vi "SolveFastPath.vi"(8 "error in (no error)":errorcluster, 11 "RouteTree in":refnum<class "RouteTree.lvclass">) -> (0 "error out":errorcluster, 2 "greedy Path":T1[](array[typedef]), 3 "RouteTree out":refnum<class "RouteTree.lvclass">)   [LabVIEW 2010, in "RouteTree.lvclass"]
uses:
  RouteTree.lvclass
  Waypoint/point.ctl
  Waypoint/Waypoint.lvclass
  Tree/Tree.lvclass
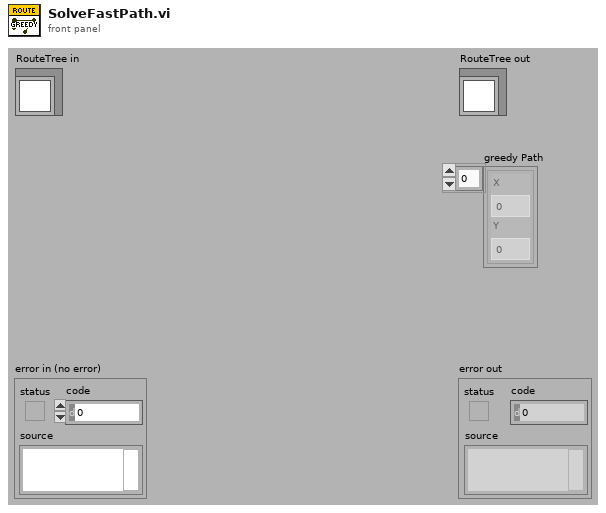
[diagram p1: front panel]
types:
  T1 = typedef "Waypoint.lvclass/point.ctl" = cluster{"X":dbl, "Y":dbl}
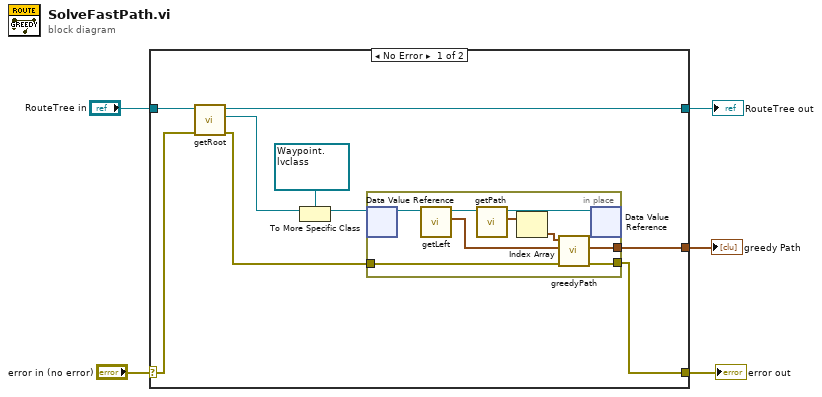
[diagram p0: block diagram]
diagram:
  n1 = case shown="No Error" "error in (no error)" {
    selector: "error in (no error)" -> [w12 w25]
    tunnel: [w7 w25] -> w4
    tunnel: [w13 w24] -> w2
    tunnel: "RouteTree in" -> [w14 w24]
    tunnel: [w6 _] -> w1
    frame No Error {
      n2 = call "getRoot.vi"("error in (no error)"=w12, "Tree in"=w14) -> ("error out"=w8:errorcluster, "Root"=w10:refnum<data-value>, "Tree out"=w13:refnum<class "RouteTree.lvclass">)  [unwired: 7 in]
      n3 = To More Specific Class(target class=refnum<data-value> refnum ("data value reference"), reference=w10) -> (specific class reference=w9:refnum<data-value>)  [unwired: 1 in, 1 out]
      n4 = in-place {
        in-place-border: [w17] -> w6
        in-place-border: w8 -> [w16]
        in-place-border: [w15] -> w7
        n5 = in-place-dvr #1(w9) -> (w23:refnum<class "Waypoint.lvclass">)  [unwired: 1 out]
        n6 = call "getLeft.vi"("Waypoint in"=w23) -> ("left"=w22:T1[], "Waypoint out"=w21:refnum<class "Waypoint.lvclass">)  [unwired: 8 in, 1 out]
        n7 = call "getPath.vi"("Waypoint in"=w21) -> ("Path"=w20:T1[], "Waypoint out"=w19:refnum<class "Waypoint.lvclass">)  [unwired: 8 in, 1 out]
        n8 = Index Array(array=w20) -> (element=w18:T1)  [unwired: 1 in]
        n9 = call "greedyPath.vi"("error in (no error)"=w16, "ToVisit"=w22, "start"=w18) -> ("error out"=w15:errorcluster, "greedy Path"=w17:T1[])  [unwired: 7 in]
        n10 = in-place-dvr #1(w19) -> ()  [unwired: 2 out]
      }
    }
    frame Error {
    }
  }
  "error out" <- w4
  "RouteTree out" <- w2
  "greedy Path" <- w1
